vi "default subpanel.vi"(10 "EVENT":refnum<user-event>, 11 "DVR":refnum<data-value>) -> ()   [LabVIEW 2013, in "VI modification.lvclass"]
uses:
  VI modification.lvclass
  VI modification.lvclass/VI modification.ctl
  Read exclusions.vi
panel:
  in  "exclusions":string[](array[string])
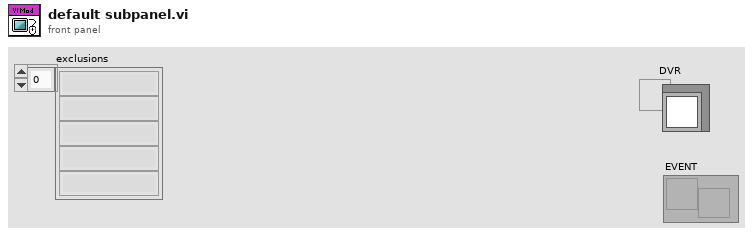
[diagram p1: front panel]
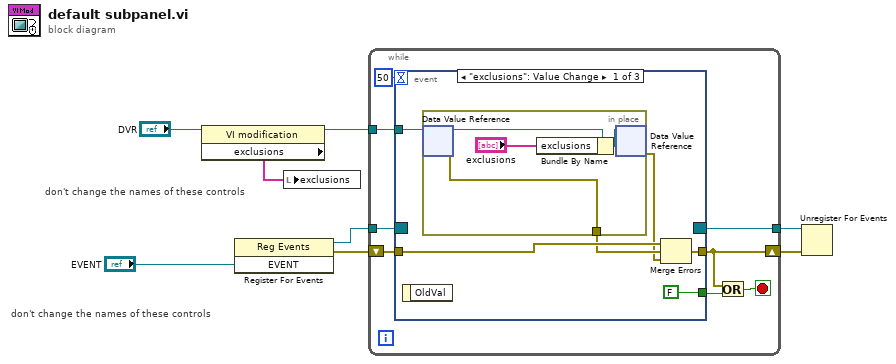
[diagram p0: block diagram]
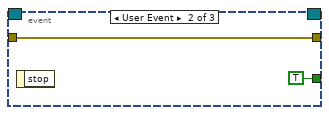
[diagram p2: hidden frame]
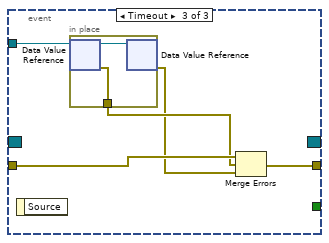
[diagram p3: hidden frame]
diagram:
  # "don't change the names of these controls"
  # "don't change the names of these controls"
  n1 = property class="VI modification"(reference="DVR") -> (reference out=w2:refnum<data-value>, "exclusions"=w1:string[])  [unwired: 1 in, 1 out]
  n2 = register-events("EVENT") -> (reference out=w6:refnum<event-registration>, error out=w7:errorcluster)  [unwired: 2 in]
  n3 = local write "exclusions"(w1) -> ()
  n4 = while {
    shift-right: [w9] -> w5
    shift-left: w7 -> [w13]
    tunnel: w6 -> [w16]
    tunnel: [w15] -> w4
    tunnel: w2 -> [w12]
    stop <- w10 stop-if-true
    n5 = event shown="[0] \"exclusions\": Value Change" {
      selector: w16 -> [_ _ _]
      dyn-events: [_ _ _] -> w15
      timeout: 50 -> [_ _ _]
      tunnel: [FALSE TRUE _] -> w14
      tunnel: [w20 w28 w31] -> w9
      tunnel: w13 -> [w22 w28 w33]
      tunnel: w12 -> [w21 _ w32]
      event "exclusions": Value Change {
        n6 = event-data() -> ()  [unwired: 1 in, 1 out]
        n7 = in-place {
          in-place-border: [w23] -> w18
          n8 = in-place-dvr #1(w21) -> (w26:refnum<class "VI modification.lvclass">, w23:errorcluster)
          n9 = Bundle By Name(cluster=w26, "exclusions"="exclusions") -> (w25:refnum<class "VI modification.lvclass">)
          n10 = in-place-dvr #1(w25) -> (w17:errorcluster)  [unwired: 1 out]
        }
        n11 = Merge Errors(w22, w18, w17) -> (w20:errorcluster)
      }
      event User Event {
        n12 = event-data() -> ()  [unwired: 1 in, 1 out]
      }
      event Timeout {
        n13 = event-data() -> ()  [unwired: 1 in, 1 out]
        n14 = in-place {
          in-place-border: [w34] -> w30
          n15 = in-place-dvr #2(w32) -> (w35:refnum<class "VI modification.lvclass">, w34:errorcluster)
          n16 = in-place-dvr #2(w35) -> (w29:errorcluster)  [unwired: 1 out]
        }
        n17 = Merge Errors(w33, w30, w29) -> (w31:errorcluster)
      }
    }
    n18 = Or(x=w9, y=w14) -> (x .or. y?=w10:bool)
  }
  n19 = Unregister For Events(event registration refnum=w4, error in=w5) -> ()  [unwired: 1 out]
